vi "RSZVB Trace Diagram Area Catalog.vi"(8 "error in (no error)":errorcluster {"code" format="%.0x"}, 10 "Window (1)":i32=1, 11 "VISA session":refnum<visa-resource-name>) -> (0 "error out":errorcluster {"code" format="%.0x"}, 2 "Catalog":string, 3 "dup VISA session":refnum<visa-resource-name>)   [LabVIEW 2011]
doc: "This VI returns the numbers and names of all traces in diagram area no. <Wnd>. \n\nRemote-control command(s):\nDISPlay[:WINDow<Wnd>]:TRACe<WndTr>:CATalog?"
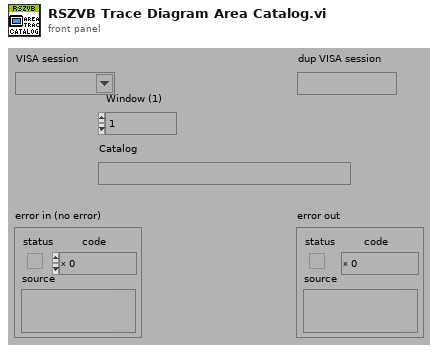
[diagram p1: front panel]
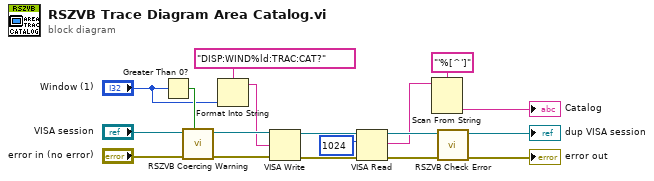
[diagram p0: block diagram]
diagram:
  n1 = Greater Than 0?(x="Window (1)") -> (x > 0?=w11:bool)
  n2 = call "RSZVB Coercing Warning.vi"("In Range?"=w11, "error in (no error)"="error in (no error)", "VISA session"="VISA session") -> ("error out"=w10:errorcluster, "dup VISA session"=w9:refnum<visa-resource-name>)  [unwired: 7 in]
  n3 = Format Into String(format string="DISP:WIND%ld:TRAC:CAT?", "Window (1)") -> (resulting string=w7:string)  [unwired: 2 in, 1 out]
  n4 = VISA Write(VISA resource name=w9, write buffer=w7, error in (no error)=w10) -> (VISA resource name out=w17:refnum<visa-resource-name>, error out=w16:errorcluster)  [unwired: 1 out]
  n5 = VISA Read(VISA resource name=w17, byte count=u32 1024 ("byte count (0)"), error in (no error)=w16) -> (VISA resource name out=w15:refnum<visa-resource-name>, read buffer=w13:string, error out=w14:errorcluster)  [unwired: 1 out]
  n6 = Scan From String(format string="'%[^']", input string=w13) -> (output 1=→"Catalog":string)  [unwired: 3 in, 3 out]
  n7 = call "RSZVB Check Error.vi"("error in (no error)"=w14, "VISA session"=w15) -> ("error out"=→"error out":errorcluster, "dup VISA session"=→"dup VISA session":refnum<visa-resource-name>)  [unwired: 8 in]
